vi "TF_Tacho2Velocity.vi"(0 "Action (Read)":T2=enum."Read", 2 "Motor Velocity Tacho Value [V]":dbl, 3 "ETH Mike Model":T1) -> (5 "Motor Velocity Tacho [deg/s]":dbl)   [LabVIEW 2019]
uses:
  ReadOnlyGlobalActions.ctl
  ETHMikeModel.ctl
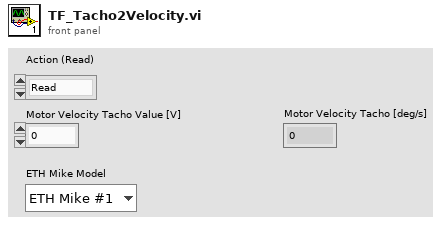
[diagram p1: front panel]
types:
  T1 = typedef "ETHMikeModel.ctl" = enum16{"ETH Mike #1", "ETH Mike #2", "ETH Mike #3", "ETH Mike #4", "ETH MIKE #5"}
  T2 = typedef "ReadOnlyGlobalActions.ctl" = enum16{"Initialize", "Read"}
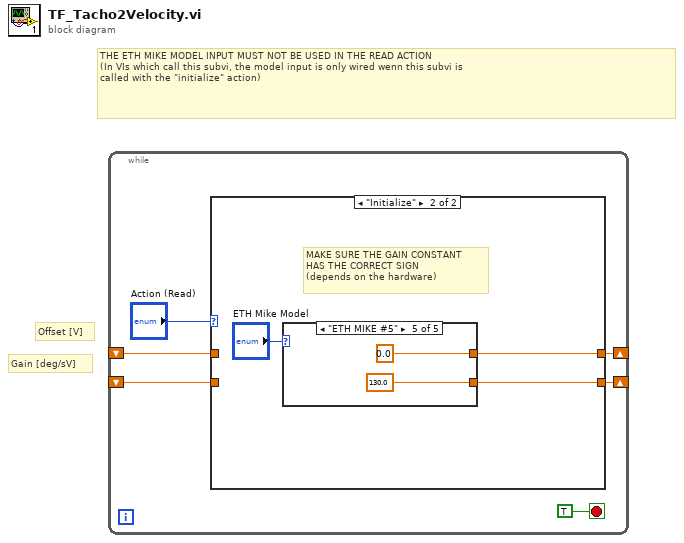
[diagram p0: block diagram]
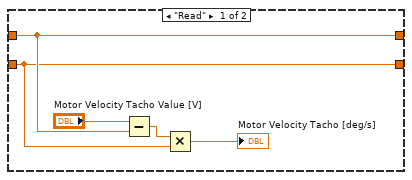
[diagram p2: hidden frame]
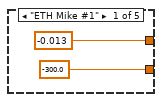
[diagram p3: hidden frame]
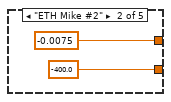
[diagram p4: hidden frame]
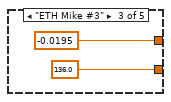
[diagram p5: hidden frame]
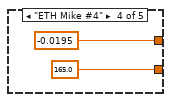
[diagram p6: hidden frame]
diagram:
  # "THE ETH MIKE MODEL INPUT MUST NOT BE USED IN THE READ ACTION\n(In VIs which call this subvi, the model input is only wired wenn this subvi is\ncalled with the \"initialize\" action)"
  # "Gain [deg/sV]"
  # "Offset [V]"
  n1 = while {
    shift-right: [w5] -> _
    shift-left: _ -> [w4]
    shift-right: [w2] -> _
    shift-left: _ -> [w1]
    stop <- TRUE stop-if-true
    n2 = case shown="\"Initialize\"" "Action (Read)" {
      tunnel: [w10 w13] -> w5
      tunnel: w4 -> [w10 _]
      tunnel: [w8 w12] -> w2
      tunnel: w1 -> [w8 _]
      frame "Read" {
        n3 = Subtract(x="Motor Velocity Tacho Value [V]", y=w10) -> (x-y=w9:dbl)
        n4 = Multiply(x=w9, y=w8) -> (x*y=→"Motor Velocity Tacho [deg/s]":dbl)
      }
      frame "Initialize" {
        # "MAKE SURE THE GAIN CONSTANT\nHAS THE CORRECT SIGN \n(depends on the hardware)"
        n5 = case shown="\"ETH MIKE #5\"" "ETH Mike Model" {
          tunnel: [-0.013 ("Offset [V]") -0.0075 ("Offset [V]") -0.0195 ("Offset [V]") -0.0195 ("Offset [V]") 0.0 ("Offset [V]")] -> w13
          tunnel: [-300.0 ("Gain [deg/sV]") -400.0 ("Gain [deg/sV]") 136.0 ("Gain [deg/sV]") 165.0 ("Gain [deg/sV]") 130.0 ("Gain [deg/sV]")] -> w12
          frame "ETH Mike #1" {
          }
          frame "ETH Mike #2" {
          }
          frame "ETH Mike #3" {
          }
          frame "ETH Mike #4" {
          }
          frame "ETH MIKE #5" {
          }
        }
      }
    }
  }
